vi "testScriptCompiler.vi"(10 "Path":path) -> ()   [LabVIEW 2009, in "run.lvlib"]
uses:
  run.lvlib
  Tools/DatabaseHelpers/DbConnection/DeviceDataBase/deviceDataBase.lvclass
  Channels/Digital/DigitalOutput.lvclass
  Channels/VoltOutput/AnalogOutput.lvclass
  Channels/DDSOutput/Generic/DDSOutput.lvclass
  Tools/Filing/FileNeologist/FileNeologist.lvclass
  Tools/DataMappers/DeviceData/DeviceData.lvclass
  Tools/DataMappers/DeviceData/DoDeviceData/DoDeviceData.lvclass
  Tools/DataMappers/DeviceData/AoDeviceData/AoDeviceData.lvclass
  Tools/DataMappers/DeviceData/RfOutputData/RfOutputData.lvclass
  Tools/SettingsProcessors/ScriptListCompiler/ScriptListCompiler.lvclass
  Tools/DatabaseHelpers/Database Objects/DeviceArray/DeviceArray.lvclass
  Tools/DatabaseHelpers/Database Objects/device/device.lvclass
  Tools/Scripting/ScriptingEvent/ScriptEventList/ScriptEventList.lvclass
  Tools/Filing.lvlib
panel:
  out "database out":refnum<class "deviceDataBase.lvclass">
  out "DB":dbl format="%_9g"
  out "error out":errorcluster
  out "rfDataArray":cluster{dbl[][]}[](array[cluster])
  out "rf physicalChannels":string[](array[string])
  in  "Channel Nr":i32
  out "timingDo":dbl
  out "timingAO":dbl
  out "compiler":dbl
  out "eventStringArray":string[][][](array[string])
  out "digital Data":T1 {"Timestamps ms" format="%#_10g"}
  out "Timing 2":T2
  out "analog data":dbl[][](array[numeric])
  out "Ranges":dbl[](array[numeric])
  out "Physical Channels 2":string
  out "Digital":string
  out "Routings":cluster{"Master Clock Route":string[]}
  out "Timing":T3
  out "Physical Channels":string
  out "AO channel":string
  out "timing":dbl
  # "time does not include\nopen database\ntime"
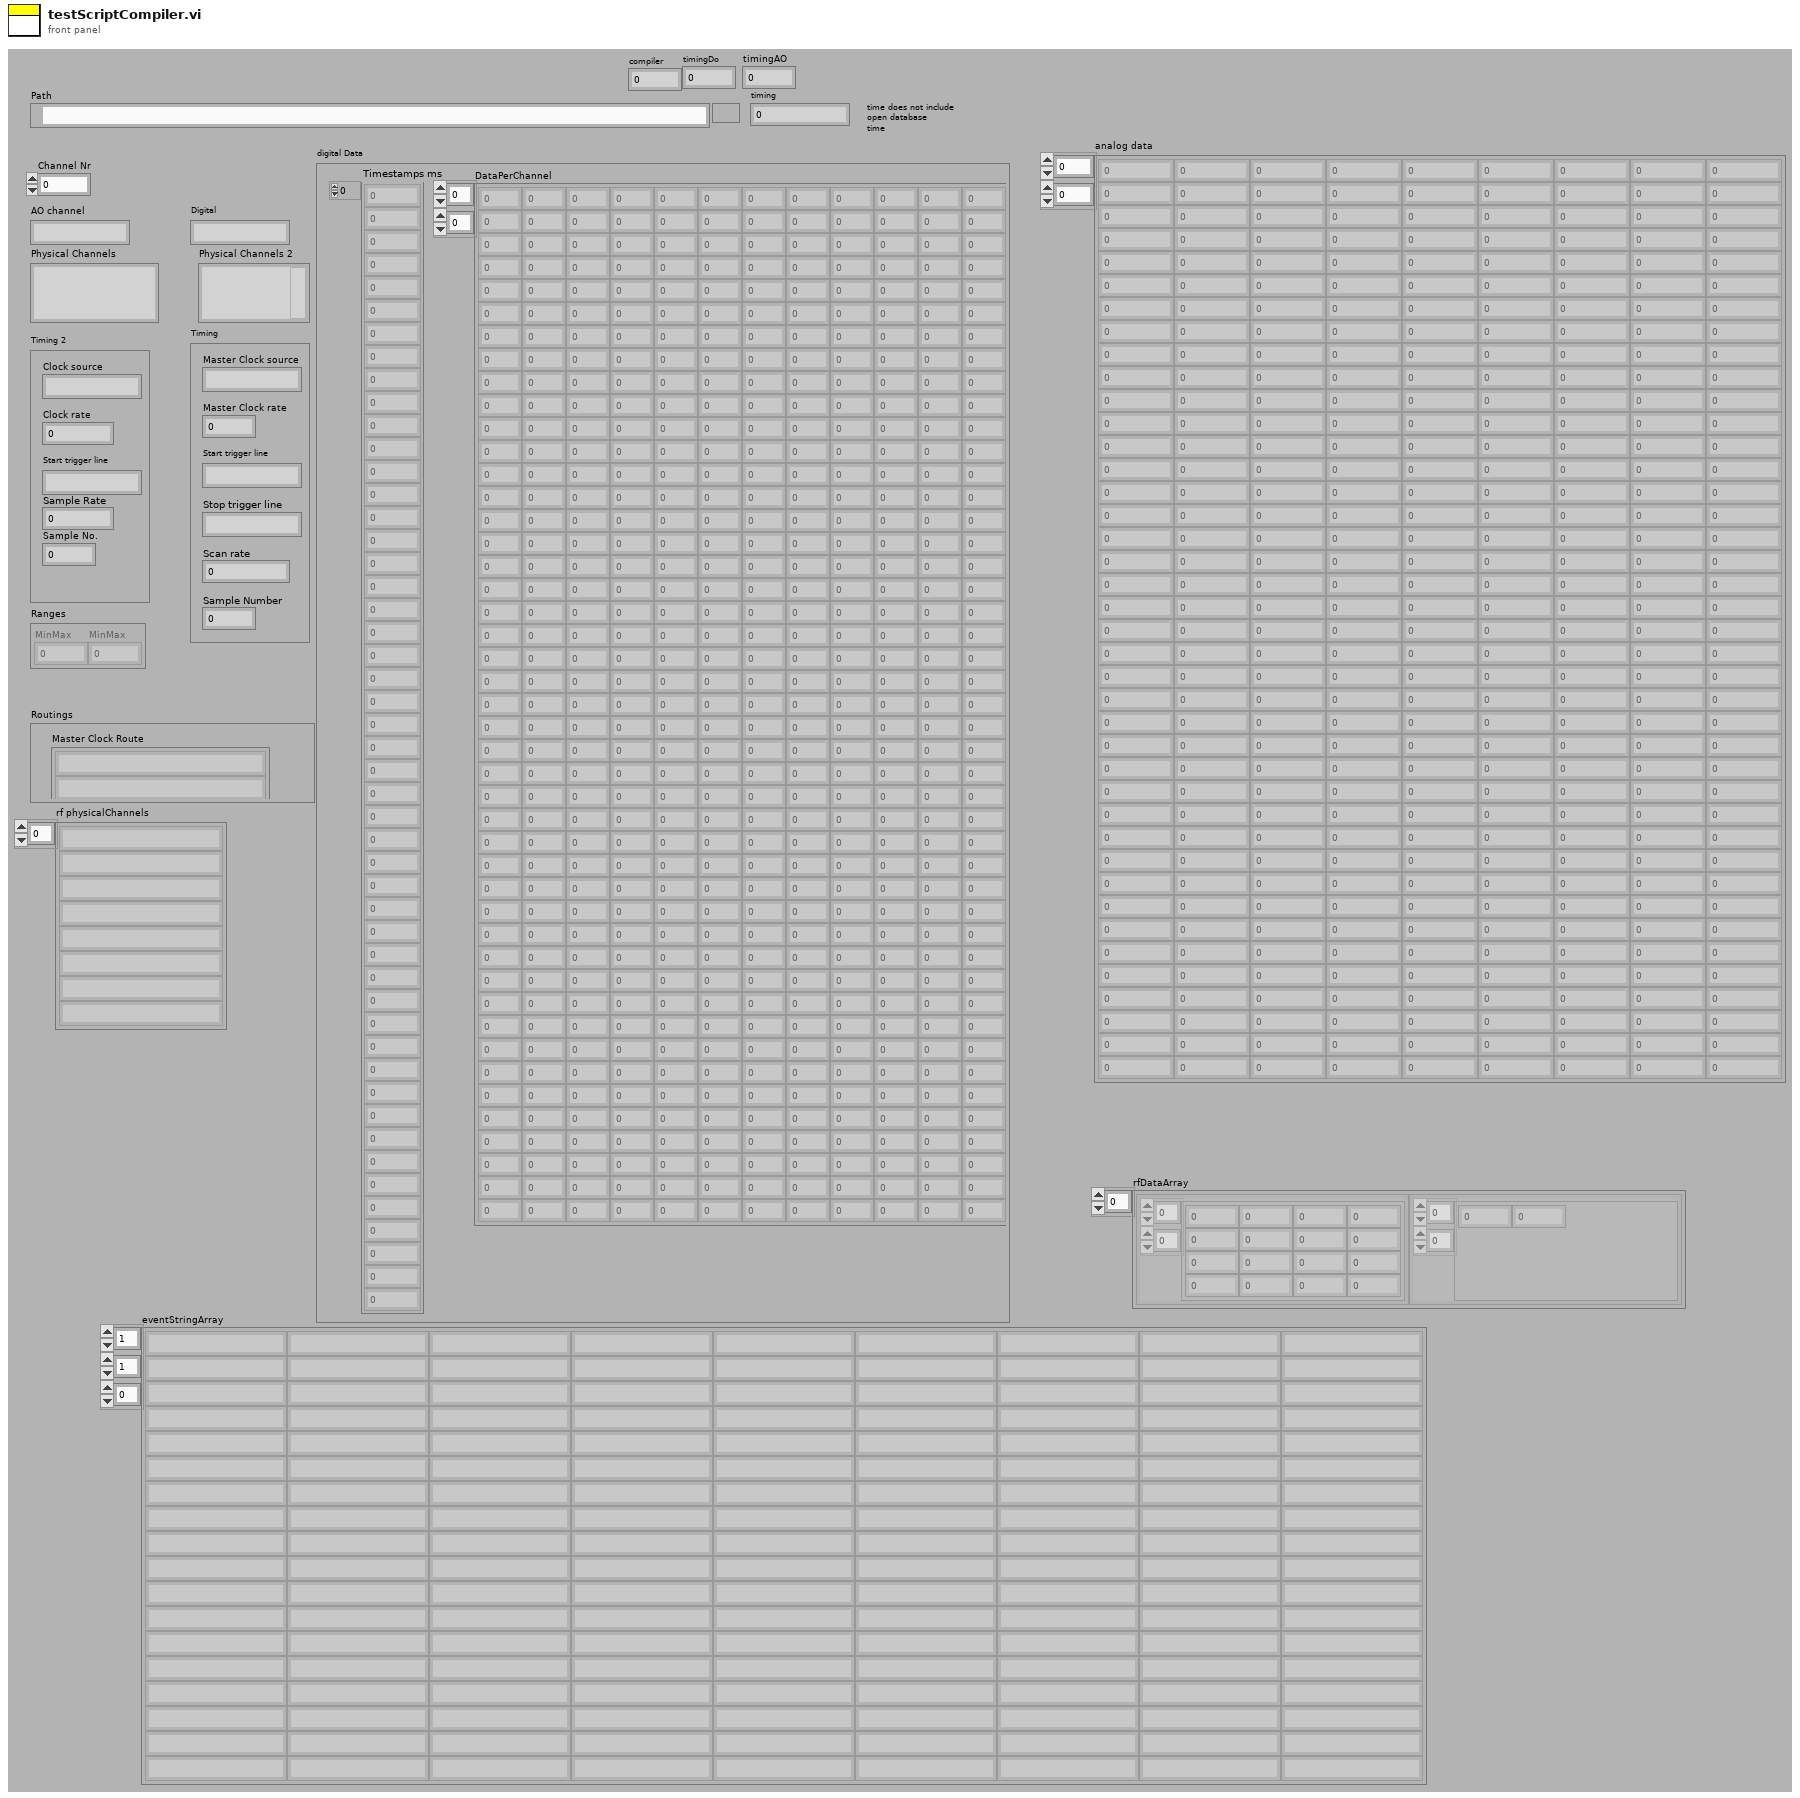
[diagram p1: front panel]
types:
  T1 = cluster{"Timestamps ms":dbl[], "DataPerChannel":dbl[][]}
  T2 = cluster{"Clock source":string, "Clock rate":dbl, "Start trigger line":string, "Sample Rate":dbl, "Sample No.":dbl}
  T3 = cluster{"Master Clock source":string, "Master Clock rate":dbl, "Start trigger line":string, "Scan rate":dbl, "Stop trigger line":string, "Sample Number":dbl}
  T4 = enum16{"digitalOutput", "digitalInput", "analogOutput", "analogInput", "rfOutput", "ethernetSupply"}
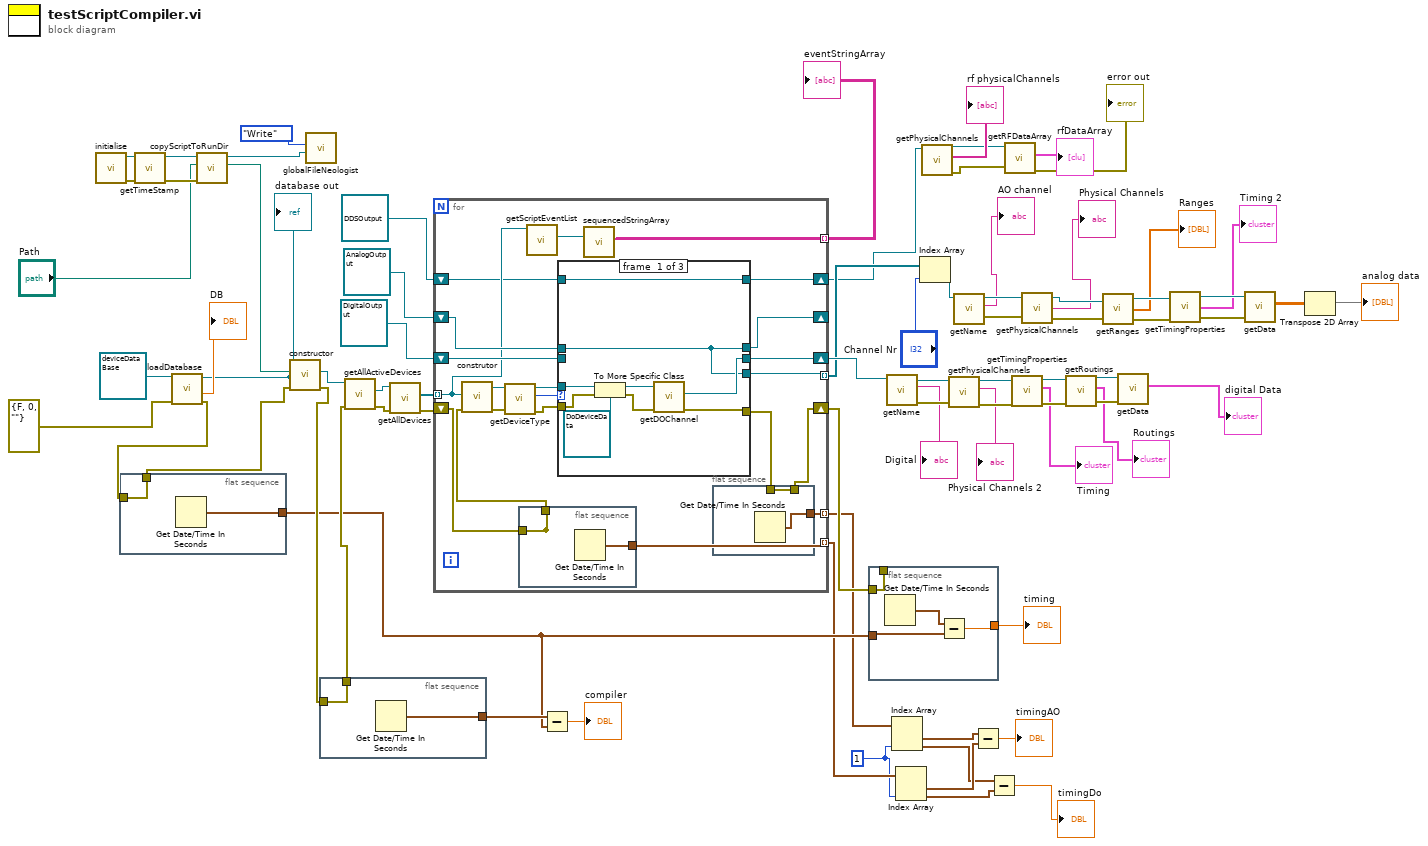
[diagram p0: block diagram]
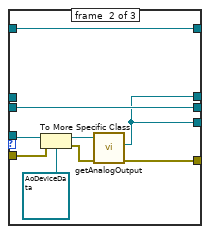
[diagram p2: hidden frame]
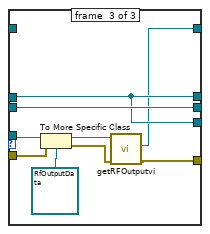
[diagram p3: hidden frame]
diagram:
  w46 = 1
  n1 = call "initialise.vi"() -> ("error out"=w70:errorcluster, "FileNeologist out"=w69:refnum<class "FileNeologist.lvclass">)  [unwired: 10 in]
  n2 = flat-sequence {
    tunnel: [w78] -> w54
    tunnel: w12 -> [w77]
    tunnel: [w77] -> w11
    frame #0 {
      n3 = Get Date/Time In Seconds() -> (seconds since 1Jan1904=w78:timestamp)
    }
  }
  n4 = call "getTimeStamp.vi"("error in (no error)"=w70, "FileNeologist in"=w69) -> ("error out"=w68:errorcluster, "FileNeologist out"=w67:refnum<class "FileNeologist.lvclass">)  [unwired: 7 in, 1 out]
  n5 = call "loadDatabase.vi"("error in (no error)"=errorcluster {"status"=FALSE, "code"=0, "source"=""}, "deviceDataBase in"=refnum<class "deviceDataBase.lvclass"> refnum) -> ("error out"=w12:errorcluster, "total"=→"DB":dbl, "deviceDataBase out"=w2:refnum<class "deviceDataBase.lvclass">)  [unwired: 7 in]
  "database out" <- w2
  n6 = call-dynamic "copyScriptToRunDir.vi"("error in (no error)"=w68, "Path in"="Path", "FileNeologist in"=w67) -> ("Path out"=w66:path, "FileNeologist out"=w58:refnum<class "FileNeologist.lvclass">)  [unwired: 6 in, 1 out]
  n7 = call "constructor.vi"("error in (no error)"=w11, "deviceDataBase"=w2, "Path"=w66) -> ("error out"=w57:errorcluster, "DeviceArray"=w65:refnum<class "DeviceArray.lvclass">)  [unwired: 5 in, 2 out]
  n8 = call "globalFileNeologist.vi"("FileNeologist in"=w58, "Action"=enum16{"Write", "Read"}."Write") -> ()  [unwired: 9 in, 1 out]
  n9 = flat-sequence {
    tunnel: [w80] -> w55
    tunnel: w57 -> [w79]
    tunnel: [w79] -> w56
    frame #0 {
      n10 = Get Date/Time In Seconds() -> (seconds since 1Jan1904=w80:timestamp)
    }
  }
  n11 = call "getAllActiveDevices.vi"("error in (no error)"=w56, "DeviceArray in"=w65) -> ("error out"=w64:errorcluster, "DeviceArray"=w63:refnum<class "DeviceArray.lvclass">)  [unwired: 7 in, 1 out]
  n12 = call "getAllDevices.vi"("error in (no error)"=w64, "DeviceArray.lvclass in"=w63) -> ("error out"=w61:errorcluster, "deviceArray"=w62:refnum<class "device.lvclass">[])  [unwired: 7 in, 1 out]
  n13 = for {
    shift-right: [w85] -> w72
    shift-left: w61 -> [w89]
    shift-right: [w97] -> w71
    shift-left: refnum<class "DigitalOutput.lvclass"> refnum ("DigitalOutput") -> [w96]
    shift-right: [w95] -> _
    shift-left: refnum<class "AnalogOutput.lvclass"> refnum ("aOChannel") -> [w94]
    tunnel: w62 -> [w91] mode=indexing
    tunnel: [w90] -> w60 mode=indexing
    tunnel: [w87] -> w51 mode=indexing
    tunnel: [w84] -> w52 mode=indexing
    tunnel: [w83] -> w16 mode=indexing
    shift-right: [w81] -> w9
    shift-left: refnum<class "DDSOutput.lvclass"> refnum ("Hardware:Channels.lvlib:DDSOutput.lvclass") -> [w82]
    n14 = call "construtor.vi"("error in (no error)"=w88, "device"=w91) -> ("error out"=w101:errorcluster, "DeviceData out"=w100:refnum<class "DeviceData.lvclass">)  [unwired: 8 in]
    n15 = call-dynamic "getDeviceType.vi"("error in (no error)"=w101, "DeviceData in"=w100) -> ("error out"=w93:errorcluster, "type"=w99:T4, "DeviceData out"=w98:refnum<class "DeviceData.lvclass">)  [unwired: 7 in]
    n16 = flat-sequence {
      tunnel: [w105] -> _
      tunnel: [w105] -> w88
      tunnel: w89 -> [w105]
      tunnel: [w104] -> w87
      frame #0 {
        n17 = Get Date/Time In Seconds() -> (seconds since 1Jan1904=w104:timestamp)
      }
    }
    n18 = call "getScriptEventList.vi"("device.lvclass in"=w91) -> ("ScriptEventList"=w92:refnum<class "ScriptEventList.lvclass">)  [unwired: 8 in, 2 out]
    n19 = case shown="\"rfOutput\"" w99 {
      tunnel: w98 -> [w114 w122 w132]
      tunnel: [w111 w119 w131] -> w97
      tunnel: w96 -> [_ w119 w131]
      tunnel: [w107 w116 w125] -> w95
      tunnel: w94 -> [w107 _ w125]
      tunnel: w93 -> [w110 w118 w130]
      tunnel: [w108 w117 w126] -> w86
      tunnel: [w107 w116 w125] -> w83
      tunnel: w82 -> [w106 w115 _]
      tunnel: [w106 w115 w124] -> w81
      frame #0 {
        n20 = To More Specific Class(target class=refnum<class "DoDeviceData.lvclass"> refnum ("DoDeviceData.lvclass in"), reference=w114, error in=w110) -> (specific class reference=w112:refnum<class "DoDeviceData.lvclass">, error out=w109:errorcluster)
        n21 = call "getDOChannel.vi"("error in (no error)"=w109, "DoDeviceData.lvclass in"=w112) -> ("error out"=w108:errorcluster, "DigitalOutput"=w111:refnum<class "DigitalOutput.lvclass">)  [unwired: 7 in, 1 out]
      }
      frame #1 {
        n22 = To More Specific Class(target class=refnum<class "AoDeviceData.lvclass"> refnum ("AoDeviceData.lvclass in"), reference=w122, error in=w118) -> (specific class reference=w120:refnum<class "AoDeviceData.lvclass">, error out=w123:errorcluster)
        n23 = call "getAnalogOutput.vi"("error in (no error)"=w123, "AoDeviceData.lvclass in"=w120) -> ("error out"=w117:errorcluster, "aOChannel"=w116:refnum<class "AnalogOutput.lvclass">)  [unwired: 7 in, 1 out]
      }
      frame #2 {
        n24 = To More Specific Class(target class=refnum<class "RfOutputData.lvclass"> refnum ("DataMappers.lvlib:RfOutputData.lvclass"), reference=w132, error in=w130) -> (specific class reference=w128:refnum<class "RfOutputData.lvclass">, error out=w127:errorcluster)
        n25 = call-dynamic "getRFOutputvi.vi"("error in (no error)"=w127, "RfOutputData in"=w128) -> ("error out"=w126:errorcluster, "DDSOutput"=w124:refnum<class "DDSOutput.lvclass">)  [unwired: 7 in, 1 out]
      }
    }
    n26 = call "sequencedStringArray.vi"("ScriptEventList in"=w92) -> ("eventStringArray"=w90:string[][])  [unwired: 8 in, 2 out]
    n27 = flat-sequence {
      tunnel: [w103] -> w84
      tunnel: w86 -> [w102]
      tunnel: [w102] -> _
      tunnel: [w102] -> w85
      frame #0 {
        n28 = Get Date/Time In Seconds() -> (seconds since 1Jan1904=w103:timestamp)
      }
    }
  }
  "eventStringArray" <- w60
  n29 = Subtract(x=w55, y=w54) -> (x-y=→"compiler":dbl)
  n30 = flat-sequence {
    tunnel: w54 -> [w135]
    tunnel: [w134] -> w75
    tunnel: w72 -> [w133]
    tunnel: [w133] -> _
    frame #0 {
      n31 = Get Date/Time In Seconds() -> (seconds since 1Jan1904=w136:timestamp)
      n32 = Subtract(x=w136, y=w135) -> (x-y=w134:dbl)
    }
  }
  n33 = call-dynamic "getName.vi"("DigitalOutput.lvclass in"=w71) -> ("error out"=w29:errorcluster, "name"=→"Digital":string, "DigitalOutput.lvclass out"=w30:refnum<class "DigitalOutput.lvclass">)  [unwired: 8 in]
  n34 = Index Array(array=w52, index #2=w46) -> (element #1=w50:timestamp, element #2=w48:timestamp)  [unwired: 1 in]
  n35 = Index Array(array=w51, index #2=w46) -> (element #1=w49:timestamp, element #2=w47:timestamp)  [unwired: 1 in]
  n36 = Index Array(array=w16, index="Channel Nr") -> (element=w15:refnum<class "AnalogOutput.lvclass">)
  n37 = call "getPhysicalChannels.vi"("DDSOutput in"=w9) -> ("error out"=w6:errorcluster, "physicalChannels"=→"rf physicalChannels":string[], "DDSOutput out"=w7:refnum<class "DDSOutput.lvclass">)  [unwired: 8 in]
  n38 = call-dynamic "getPhysicalChannels.vi"("error in (no error)"=w29, "DigitalOutput.lvclass in"=w30) -> ("error out"=w27:errorcluster, "Physical Channels"=→"Physical Channels 2":string, "DigitalOutput.lvclass out"=w28:refnum<class "DigitalOutput.lvclass">)  [unwired: 7 in]
  n39 = call "getName.vi"("AnalogOutput.lvclass in"=w15) -> ("error out"=w43:errorcluster, "name"=→"AO channel":string, "AnalogOutput.lvclass out"=w39:refnum<class "AnalogOutput.lvclass">)  [unwired: 8 in]
  n40 = Subtract(x=w50, y=w49) -> (x-y=→"timingAO":dbl)
  n41 = Subtract(x=w48, y=w47) -> (x-y=→"timingDo":dbl)
  n42 = call "getRFDataArray.vi"("error in (no error)"=w6, "DDSOutput in"=w7) -> ("error out"=→"error out":errorcluster, "rfDataArray"=→"rfDataArray":cluster{dbl[][]}[])  [unwired: 7 in, 1 out]
  n43 = call-dynamic "getTimingProperties.vi"("error in (no error)"=w27, "DigitalOutput.lvclass in"=w28) -> ("error out"=w25:errorcluster, "Timing"=→"Timing":T3, "DigitalOutput.lvclass out"=w26:refnum<class "DigitalOutput.lvclass">)  [unwired: 7 in]
  n44 = call-dynamic "getPhysicalChannels.vi"("AnalogOutput.lvclass in"=w39, "error in (no error)"=w43) -> ("AnalogOutput.lvclass out"=w38:refnum<class "AnalogOutput.lvclass">, "Physical Channels"=→"Physical Channels":string, "error out"=w42:errorcluster)
  n45 = call-dynamic "getRoutings.vi"("error in (no error)"=w25, "DigitalOutput.lvclass in"=w26) -> ("error out"=w23:errorcluster, "Routings"=→"Routings":cluster{"Master Clock Route":string[]}, "DigitalOutput.lvclass out"=w24:refnum<class "DigitalOutput.lvclass">)  [unwired: 7 in]
  n46 = call "getRanges.vi"("AnalogOutput.lvclass in"=w38, "error in (no error)"=w42) -> ("AnalogOutput.lvclass out"=w37:refnum<class "AnalogOutput.lvclass">, "Ranges"=→"Ranges":dbl[], "error out"=w41:errorcluster)
  n47 = call-dynamic "getData.vi"("error in (no error)"=w23, "DigitalOutput.lvclass in"=w24) -> ("Data"=→"digital Data":T1)  [unwired: 7 in, 2 out]
  n48 = call "getTimingProperties.vi"("AnalogOutput.lvclass in"=w37, "error in (no error)"=w41) -> ("AnalogOutput.lvclass out"=w36:refnum<class "AnalogOutput.lvclass">, "Timing"=→"Timing 2":T2, "error out"=w40:errorcluster)
  n49 = call "getData.vi"("error in (no error)"=w40, "AnalogOutput.lvclass in"=w36) -> ("Data"=w31:dbl[][])  [unwired: 7 in, 2 out]
  n50 = Transpose 2D Array(2D array=w31) -> (transposed array=→"analog data":dbl[][])
  "timing" <- w75
